vi "CloneMethod.vi"(0 "ClassWriterNative.lvclass":refnum<class "ClassWriterNative.lvclass">, 1 "VIItemRefIn":refnum<vi>, 2 "NewVIPath":path, 3 "LibraryOwners":refnum<vi>[](array[refnum]), 4 "OpenVIWhenDone":bool, 5 "error in (no error)":errorcluster, 7 "ViDescription":string) -> (14 "ClassWriterNative.lvclass":refnum<class "ClassWriterNative.lvclass">, 19 "error out":errorcluster)   [LabVIEW 2020, in "ClassWriterNative.lvclass"]
uses:
  ClassWriterNative.lvclass
  Provider_EndevoGOOP400/EndevoG4ProviderName.ctl
  <vilib>/picture/picture.llb/imagedata.ctl
  <vilib>/Utility/lvfile.llb/NI_FileType.lvlib
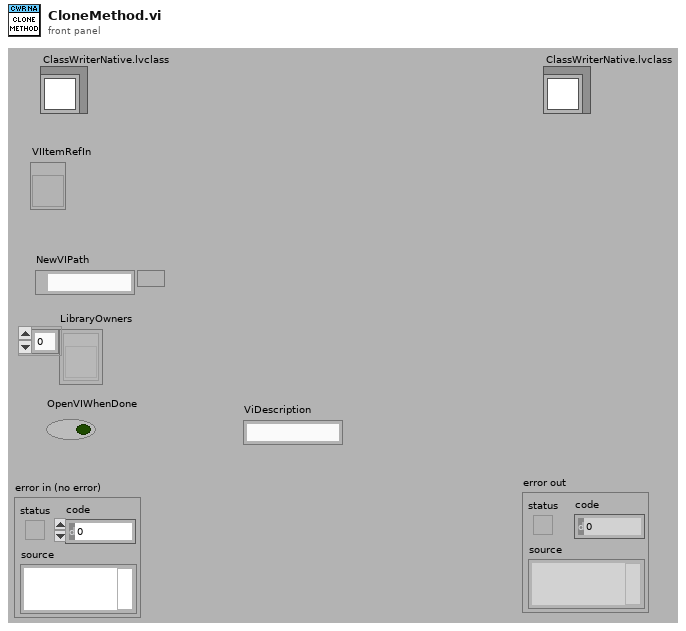
[diagram p1: front panel]
types:
  T1 = cluster{"OrgPath":path, "VIRef":refnum<vi>, "AppRef":refnum<vi>, "NewViRefs":refnum<vi>[], "VIOwner":refnum<vi>, "OrgViLibName":string, "OrgLibFolder":path, "OrgClassPath":path, "OrgClassPathMemberData":path, "FileBackups":string[], "Scope":enum32{"invalid scope", "public", "private", "protected", "community"}}
  T2 = typedef "EndevoG4ProviderName.ctl" = enum16{"EndevoGOOP400"}
  T3 = enum32{"invalid scope", "public", "private", "protected", "community"}
  T4 = typedef "imagedata.ctl" = cluster{"image type":i32, "image depth":i32, "image":u8[], "mask":u8[], "colors":u32[], "Rectangle":cluster{"left":i16, "top":i16, "right":i16, "bottom":i16}}
  T5 = typedef "GOOP400_Options.ctl" = cluster{"FlatFolderStructure":bool}
  T6 = enum32{"invalid scope", "public", "private", "protected", "community"}[]
  T7 = typedef "GDSLvClass_IconSettingsType.ctl" = cluster{"Frame":u32, "Frame thickness":u8, "Header Background":u32, "Header Text":u32, "ColorPublic":u32, "ColorProtected":u32, "ColorPrivate":u32, "Body Text":u32, "ClassBodyIcon":string}
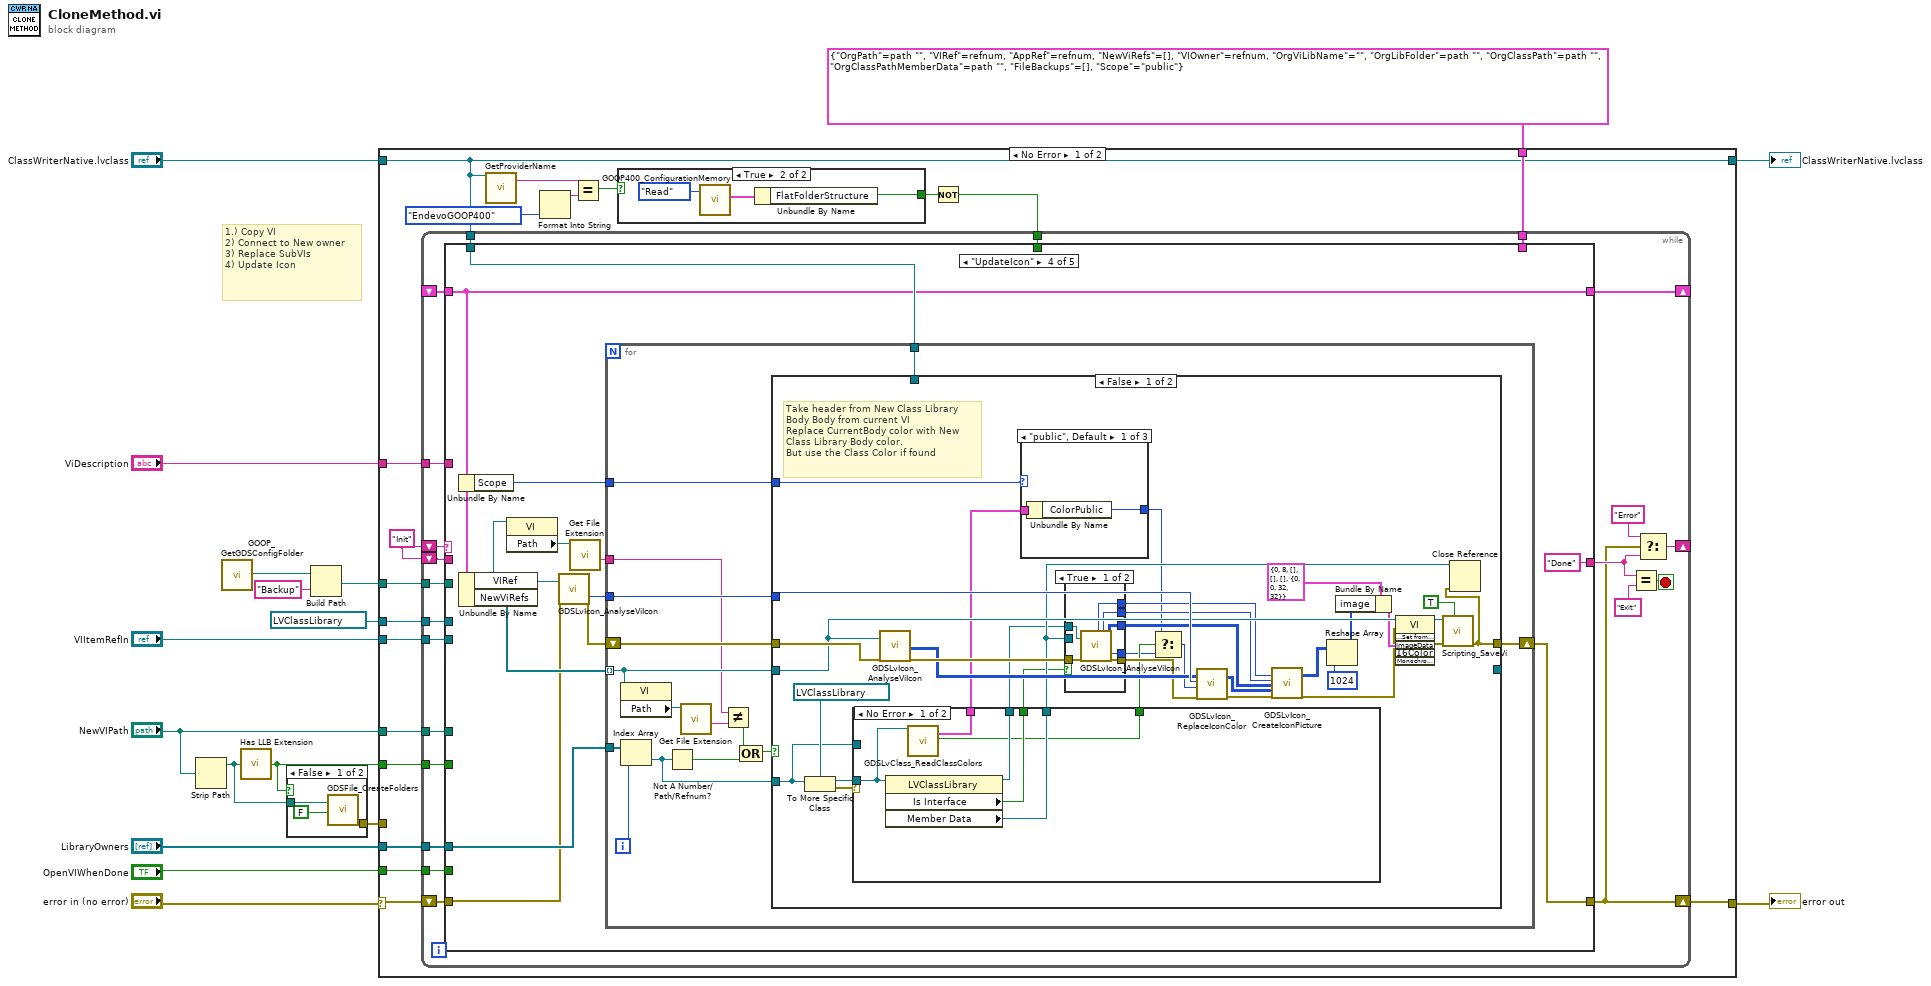
[diagram p0: block diagram]
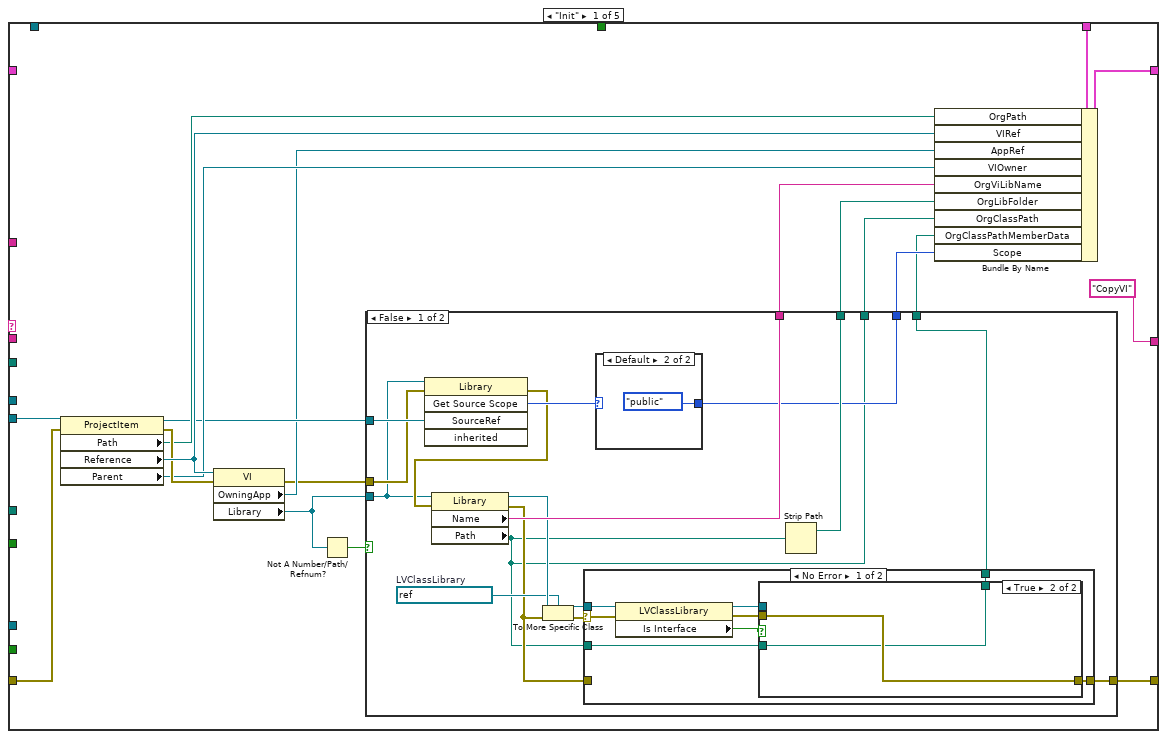
[diagram p4: hidden frame]
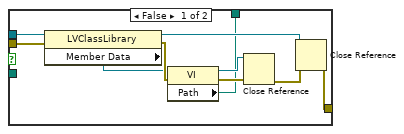
[diagram p6: hidden frame]
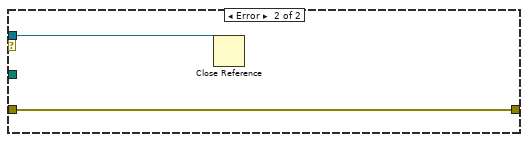
[diagram p7: hidden frame]
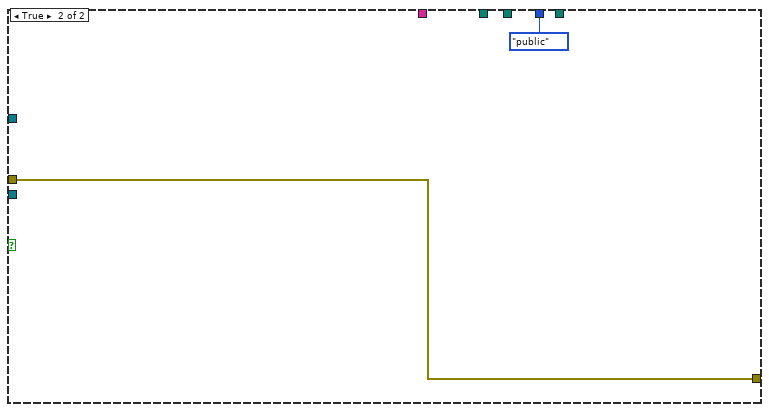
[diagram p8: hidden frame]
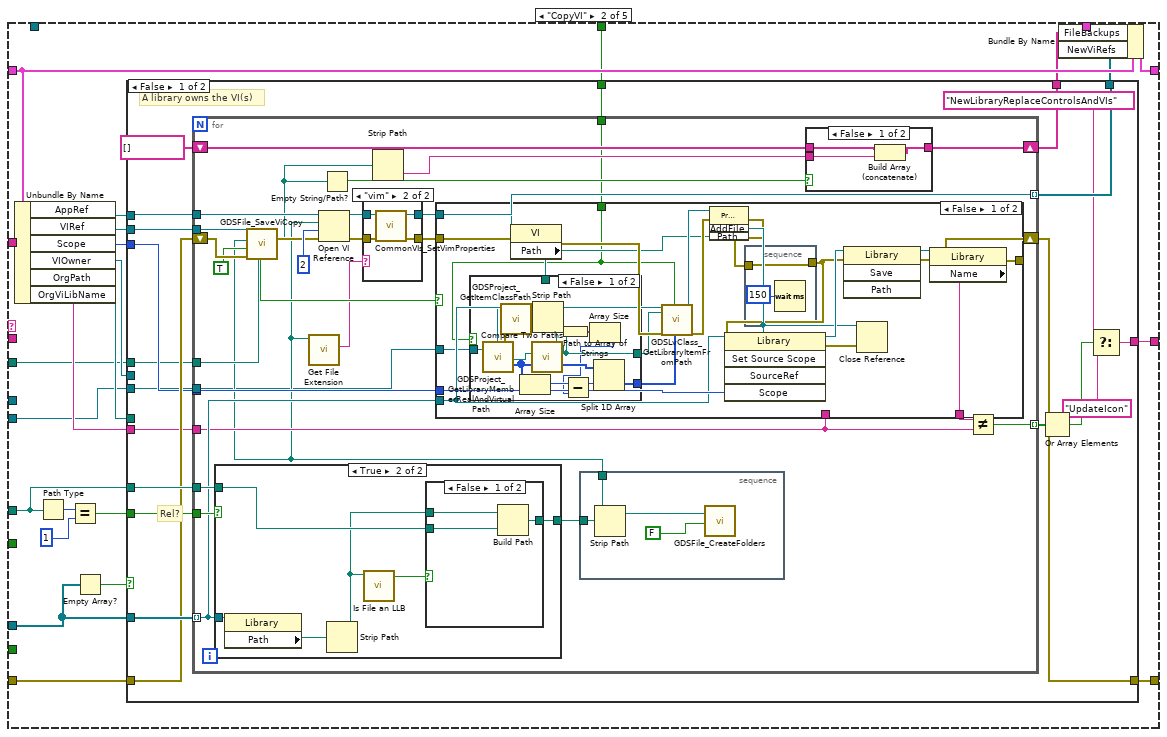
[diagram p9: hidden frame]
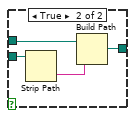
[diagram p15: hidden frame]
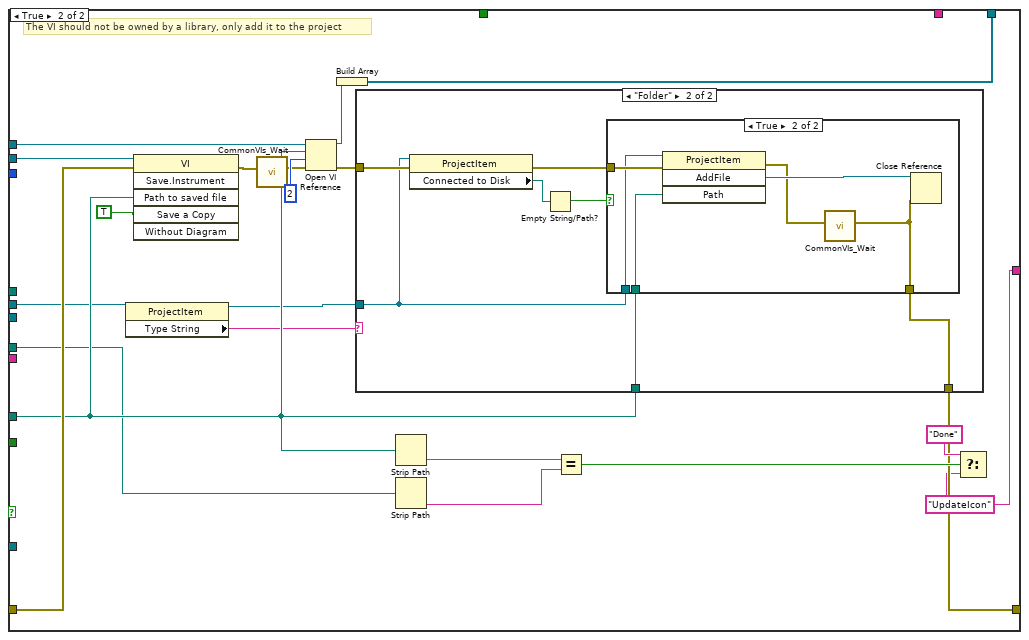
[diagram p16: hidden frame]
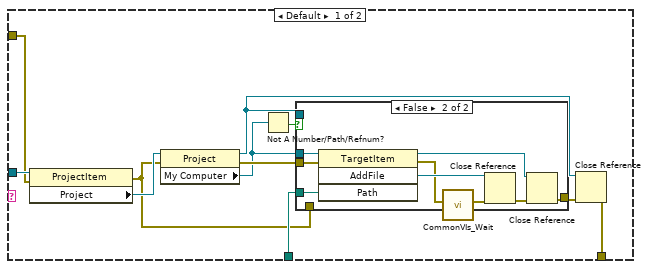
[diagram p17: hidden frame]
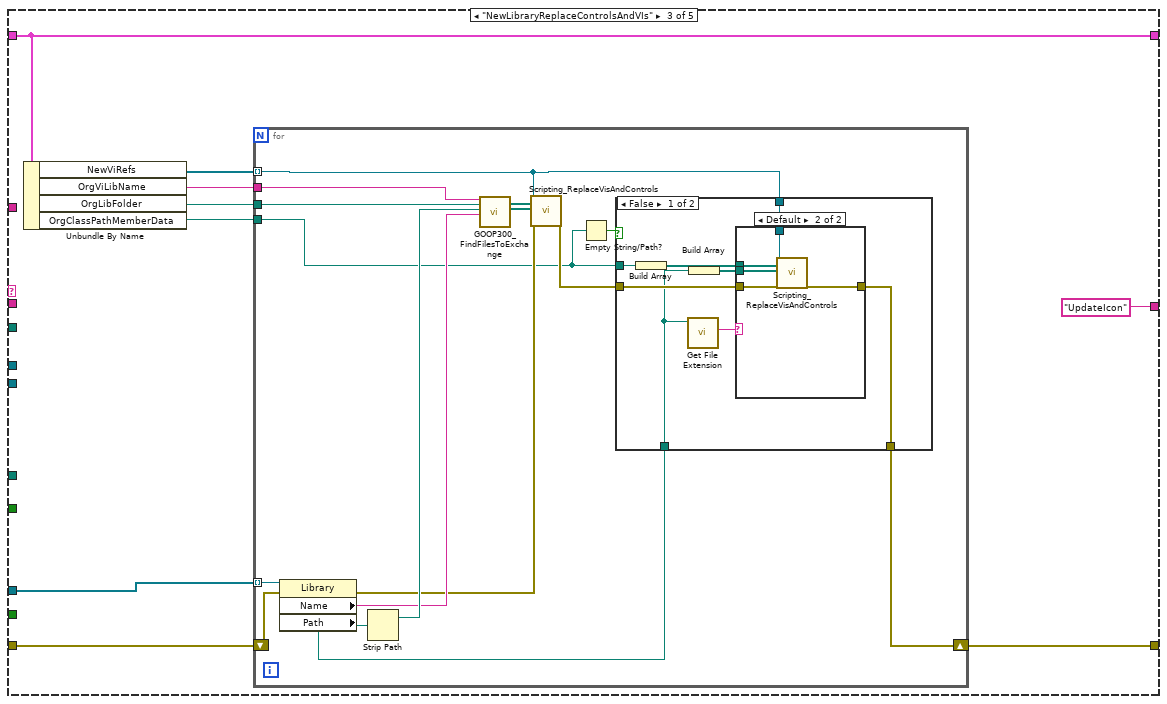
[diagram p20: hidden frame]
diagram:
  # "1.) Copy VI\n2) Connect to New owner\n3) Replace SubVIs\n4) Update Icon"
  n1 = Strip Path(path="NewVIPath") -> (stripped path=w9:path)  [unwired: 1 out]
  n2 = call "GOOP_GetGDSConfigFolder.vi"() -> ("GDSFolderPath"=w8:path)
  n3 = call <vilib>:"Has LLB Extension.vi"("path"=w9) -> ("path to VI library?"=w4:bool)
  n4 = case shown="False" w4 {
    tunnel: w9 -> [w19 _]
    tunnel: [w18 _] -> w5
    frame False {
      n5 = call "GDSFile_CreateFolders.vi"("Path"=w19, "Promt if folder\ndoes not exists?"=FALSE ("Promt if folder\ndoes not exists?")) -> ("error out"=w18:errorcluster)  [unwired: 13 in, 4 out]
    }
    frame True {
    }
  }
  n6 = Build Path(base path=w8, name or relative path="Backup") -> (appended path=w6:path)
  n7 = case shown="No Error" "error in (no error)" {
    selector: "error in (no error)" -> [w39 w529]
    tunnel: [w38 w529] -> w16
    tunnel: "ClassWriterNative.lvclass" -> [w22 w528]
    tunnel: [w22 w528] -> w14
    tunnel: refnum<vi> refnum ("ClassRefOut") -> [w37 _]
    tunnel: "NewVIPath" -> [w36 _]
    tunnel: w4 -> [w35 _]
    tunnel: "LibraryOwners" -> [w34 _]
    tunnel: "VIItemRefIn" -> [w33 _]
    tunnel: w6 -> [w32 _]
    tunnel: w5 -> [_ _]
    tunnel: "OpenVIWhenDone" -> [w31 _]
    tunnel: "ViDescription" -> [w29 _]
    tunnel: T1 {"OrgPath"=path "", "VIRef"=refnum, "AppRef"=refnum, "NewViRefs"=[], "VIOwner"=refnum, "OrgViLibName"="", "OrgLibFolder"=path "", "OrgClassPath"=path "", "OrgClassPathMemberData"=path "", "FileBackups"=[], "Scope"=enum."public"} -> [w28 _]
    frame No Error {
      w30 = "Init"
      n8 = call-dynamic "GetProviderName.vi"("ClassWriterNative in"=w22) -> ("ProviderName"=w24:string)  [unwired: 15 in, 3 out]
      n9 = Format Into String(EndevoG4ProviderName."EndevoGOOP400" ("ProviderName")) -> (resulting string=w23:string)  [unwired: 3 in, 1 out]
      n10 = Equal?(x=w24, y=w23) -> (x = y?=w26:bool)
      n11 = case shown="True" w26 {
        tunnel: [_ w40] -> w27
        frame False {
        }
        frame True {
          n12 = call "GOOP400_ConfigurationMemory.vi"("Action"=enum16{"Read", "Load", "Save"}."Read") -> ("OptionsOut"=w41:T5)  [unwired: 17 in, 1 out]
          n13 = Unbundle By Name(w41) -> ("FlatFolderStructure"=w40:bool)
        }
      }
      n14 = Not(x=w27) -> (.not. x?=w21:bool)
      n15 = while {
        shift-right: [w57] -> w38
        shift-left: w39 -> [w64]
        shift-right: [w62] -> _
        shift-left: w30 -> [w63]
        shift-right: [w56] -> _
        shift-left: _ -> [w55]
        tunnel: w37 -> [w54]
        tunnel: w36 -> [w53]
        tunnel: w35 -> [w52]
        tunnel: w34 -> [w51]
        tunnel: w33 -> [w50]
        tunnel: w32 -> [w49]
        tunnel: w22 -> [w48]
        tunnel: w31 -> [w47]
        shift-left: w30 -> [w46]
        tunnel: w29 -> [w45]
        tunnel: w28 -> [w44]
        tunnel: w21 -> [w43]
        stop <- w61 stop-if-true
        n16 = case shown="\"UpdateIcon\"" w63 {
          tunnel: w64 -> [w84 w143 w322 w367 w486]
          tunnel: [w73 w142 w321 w369 w471] -> w57
          tunnel: ["CopyVI" w139 "UpdateIcon" "Done" "Exit"] -> w58
          tunnel: [w83 w136 w327 w360 w469] -> w56
          tunnel: w55 -> [_ w137 w327 w360 w469]
          tunnel: w54 -> [_ _ _ _ _]
          tunnel: w53 -> [_ w144 _ _ _]
          tunnel: w52 -> [_ _ _ _ _]
          tunnel: w51 -> [_ w141 w325 w368 _]
          tunnel: w50 -> [w80 w127 _ _ _]
          tunnel: w49 -> [_ w130 _ _ w475]
          tunnel: w48 -> [_ _ _ w361 w474]
          tunnel: w47 -> [_ _ _ _ w473]
          tunnel: w46 -> [_ _ _ _ w470]
          tunnel: w45 -> [_ _ _ _ w468]
          tunnel: w44 -> [w65 _ _ _ _]
          tunnel: w43 -> [_ w128 _ _ _]
          frame "Init" {
            n17 = property class="ProjectItem"(reference=w80, error in=w84) -> (reference out=w72:refnum<vi>, error out=w79:errorcluster, "Path"=w75:path, "Reference"=w81:refnum<vi>, "Parent"=w78:refnum<vi>)
            n18 = property class="VI"(reference=w81, error in=w79) -> (error out=w66:errorcluster, "OwningApp"=w68:refnum<vi>, "Library"=w67:refnum<vi>)  [unwired: 1 out]
            n19 = Not A Number/Path/Refnum?(number/path/refnum=w67) -> (NaN/Path/Refnum?=w69:bool)
            n20 = case shown="False" w69 {
              tunnel: [w100 _] -> w77
              tunnel: [w99 _] -> w76
              tunnel: [w85 _] -> w74
              tunnel: [w98 w126] -> w73
              tunnel: w72 -> [w92 _]
              tunnel: [w90 T3."public" ("GetSourceScope")] -> w71
              tunnel: w66 -> [w89 w126]
              tunnel: w67 -> [w87 _]
              tunnel: [w86 _] -> w70
              frame False {
                w96 = refnum<vi> refnum  # LVClassLibrary
                n21 = invoke class="Library" method="Get Source Scope"(reference=w87, error in=w89, "SourceRef"=w92) -> (error out=w88:errorcluster, "GetSourceScope"=w91:T3)  [unwired: 2 in, 3 out]
                n22 = property class="Library"(reference=w87, error in=w88) -> (reference out=w97:refnum<vi>, error out=w94:errorcluster, "Name"=w100:string, "Path"=w85:path)
                n23 = To More Specific Class(target class=w96, reference=w97, error in=w94) -> (specific class reference=w93:refnum<vi>, error out=w95:errorcluster)
                n24 = case shown="No Error" w95 {
                  selector: w95 -> [w108 _]
                  tunnel: [w110 w124] -> w98
                  tunnel: w94 -> [_ w124]
                  tunnel: [w109 _] -> w86
                  tunnel: w93 -> [w107 w123]
                  tunnel: w85 -> [w103 _]
                  frame No Error {
                    n25 = property class="LVClassLibrary"(reference=w107, error in=w108) -> (reference out=w104:refnum<vi>, error out=w105:errorcluster, "Is Interface"=w106:bool)
                    n26 = case shown="True" w106 {
                      tunnel: [w114 w122] -> w110
                      tunnel: [w113 w121] -> w109
                      tunnel: w105 -> [w112 w122]
                      tunnel: w104 -> [w111 _]
                      tunnel: w103 -> [_ w121]
                      frame False {
                        n27 = property class="LVClassLibrary"(reference=w111, error in=w112) -> (reference out=w116:refnum<vi>, error out=w120:errorcluster, "Member Data"=w119:refnum<vi>)
                        n28 = property class="VI"(reference=w119, error in=w120) -> (reference out=w117:refnum<vi>, error out=w118:errorcluster, "Path"=w113:path)
                        n29 = Close Reference(reference=w117, error in (no error)=w118) -> (error out=w115:errorcluster)
                        n30 = Close Reference(reference=w116, error in (no error)=w115) -> (error out=w114:errorcluster)
                      }
                      frame True {
                      }
                    }
                  }
                  frame Error {
                    n31 = Close Reference(reference=w123) -> ()  [unwired: 1 in, 1 out]
                  }
                }
                n32 = case shown="Default" w91 {
                  selector: w91 -> [w101 _]
                  tunnel: [w101 T3."public" ("GetSourceScope")] -> w90
                  frame "private", "protected" {
                  }
                  frame Default {
                  }
                }
                n33 = Strip Path(path=w85) -> (stripped path=w99:path)  [unwired: 1 out]
              }
              frame True {
              }
            }
            n34 = Bundle By Name(cluster=w65, "OrgPath"=w75, "VIRef"=w81, "AppRef"=w68, "VIOwner"=w78, "OrgViLibName"=w77, "OrgLibFolder"=w76, "OrgClassPath"=w74, "OrgClassPathMemberData"=w70, "Scope"=w71) -> (w83:T1)
          }
          frame "CopyVI" {
            n35 = Unbundle By Name(w137) -> ("AppRef"=w138:refnum<vi>, "VIRef"=w145:refnum<vi>, "Scope"=w131:T3, "VIOwner"=w134:refnum<vi>, "OrgPath"=w133:path, "OrgViLibName"=w132:string)
            n36 = Path Type(1:w144) -> (0:w148:i16)
            n37 = Equal?(x=w148, y=i16 1 ("type")) -> (x = y?=w146:bool)
            n38 = Empty Array?(array=w141) -> (empty?=w140:bool)
            n39 = case shown="False" w140 {
              tunnel: w141 -> [w168 _]
              tunnel: w146 -> [w167 _]
              tunnel: w145 -> [w166 w284]
              tunnel: w144 -> [w165 w277]
              tunnel: w143 -> [w164 w278]
              tunnel: [w163 w271] -> w142
              tunnel: [w158 w267] -> w139
              tunnel: w138 -> [w162 w282]
              tunnel: [w161 w279] -> w135
              tunnel: w134 -> [_ w269]
              tunnel: w133 -> [_ w276]
              tunnel: w132 -> [w157 _]
              tunnel: w131 -> [w154 _]
              tunnel: w130 -> [w153 _]
              tunnel: [w151 _] -> w129
              tunnel: w128 -> [w150 _]
              tunnel: w127 -> [w149 _]
              frame False {
                # "A library owns the VI(s)"
                # "Rel?"
                n40 = for {
                  tunnel: w168 -> [w188] mode=indexing
                  tunnel: w167 -> [w197]
                  tunnel: w166 -> [w198]
                  tunnel: w165 -> [w196]
                  shift-right: [w189] -> w163
                  shift-left: w164 -> [w195]
                  tunnel: w162 -> [w192]
                  tunnel: [w172] -> w161 mode=indexing
                  tunnel: w157 -> [w177]
                  tunnel: [w190] -> w156 mode=indexing
                  tunnel: w154 -> [w187]
                  tunnel: w153 -> [w186]
                  shift-right: [w183] -> w151
                  shift-left: string[] [] -> [w184]
                  tunnel: w150 -> [w170]
                  tunnel: w149 -> [w169]
                  n41 = case shown="True" w197 {
                    tunnel: w188 -> [_ w256]
                    tunnel: w196 -> [w250 w254]
                    tunnel: [w250 w252] -> w179
                    frame False {
                    }
                    frame True {
                      n42 = property class="Library"(reference=w256) -> ("Path"=w255:path)  [unwired: 1 in, 2 out]
                      n43 = Strip Path(path=w255) -> (stripped path=w253:path)  [unwired: 1 out]
                      n44 = call <vilib>:"Is File an LLB.vi"("path"=w253) -> ("Is LLB?"=w251:bool)  [unwired: 9 in, 1 out]
                      n45 = case shown="False" w251 {
                        tunnel: w254 -> [w259 w261]
                        tunnel: w253 -> [w258 w262]
                        tunnel: [w257 w263] -> w252
                        frame False {
                          n46 = Build Path(base path=w258, name or relative path=w259) -> (appended path=w257:path)
                        }
                        frame True {
                          n47 = Strip Path(path=w261) -> (name=w260:string)  [unwired: 1 out]
                          n48 = Build Path(base path=w262, name or relative path=w260) -> (appended path=w263:path)
                        }
                      }
                    }
                  }
                  n49 = stacked-sequence {
                    tunnel: w179 -> [w243]
                    tunnel: [w243] -> w176
                    frame #0 {
                      n50 = Strip Path(path=w243) -> (stripped path=w244:path)  [unwired: 1 out]
                      n51 = call "GDSFile_CreateFolders.vi"("Path"=w244, "Promt if folder\ndoes not exists?"=FALSE ("Promt if folder\ndoes not exists?")) -> ()  [unwired: 13 in, 5 out]
                    }
                  }
                  n52 = call "GDSFile_SaveViCopy.vi"("BackupFolder"=w186, "error in"=w195, "OverWirite(False)"=TRUE, "NewCopyPath"=w176, "VIRef"=w198) -> ("error out"=w193:errorcluster, "OverWritten"=w178:bool, "BackupFileName"=w182:path)  [unwired: 4 in]
                  n53 = call <vilib>:"Get File Extension.vi"("file"=w176) -> ("lowercase file extension"=w171:string)  [unwired: 6 in, 4 out]
                  n54 = Open VI Reference(application reference (local)=w192, vi path=w176, options=2, error in (no error)=w193) -> (vi reference=w174:refnum<vi>, error out=w175:errorcluster)  [unwired: 2 in]
                  n55 = Empty String/Path?(string/path=w182) -> (empty?=w185:bool)
                  n56 = case shown="\"vim\"" w171 {
                    tunnel: w175 -> [w199 w204]
                    tunnel: w174 -> [w200 w203]
                    tunnel: [w199 w202] -> w173
                    tunnel: [w200 w201] -> w172
                    frame Default {
                    }
                    frame "vim" {
                      n57 = call "CommonVIs_SetVimProperties.vi"("error in (no error)"=w204, "VIRefIn"=w203) -> ("error out"=w202:errorcluster, "VIRefOut"=w201:refnum<vi>)  [unwired: 8 in]
                    }
                  }
                  n58 = Strip Path(path=w182) -> (name=w181:string)  [unwired: 1 out]
                  n59 = case shown="False" w178 {
                    tunnel: [w220 w242] -> w191
                    tunnel: w173 -> [w219 w241]
                    tunnel: w172 -> [w218 _]
                    tunnel: [w217 w241] -> w189
                    tunnel: w188 -> [w210 _]
                    tunnel: w187 -> [w213 _]
                    tunnel: w177 -> [_ w242]
                    tunnel: w170 -> [w206 _]
                    tunnel: w169 -> [w207 _]
                    frame False {
                      n60 = property class="VI"(reference=w218, error in=w219) -> (error out=w225:errorcluster, "Path"=w209:path)  [unwired: 1 out]
                      n61 = case shown="False" w206 {
                        tunnel: [w231 w238] -> w208
                        tunnel: w209 -> [_ w238]
                        tunnel: w207 -> [w237 _]
                        tunnel: [w226 _] -> w205
                        frame False {
                          n62 = call "GDSProject_GetLibraryMemberRealAndVirtualPath.vi"("LibraryItem"=w237) -> ("LibraryItemVirtualPath"=w233:path, "VirtualFolderScope"=w230:T6, "error out"=w236:errorcluster)  [unwired: 15 in, 1 out]
                          n63 = call "GDSProject_GetItemClassPath.vi"("error in"=w236, "ProjectItemRefIn"=w237) -> ("Path"=w235:path)  [unwired: 4 in, 5 out]
                          n64 = Array Size(array=w230) -> (size(s)=w229:i32)
                          n65 = Strip Path(path=w235) -> (stripped path=w234:path)  [unwired: 1 out]
                          n66 = call <vilib>:"Compare Two Paths.vi"("Path 2"=w233, "Path 1"=w234) -> ("Relative Path from 1 to 2"=w231:path)  [unwired: 6 in, 3 out]
                          n67 = Path to Array of Strings(0:w231) -> (2:w232:string[])  [unwired: 1 out]
                          n68 = Array Size(array=w232) -> (size(s)=w228:i32)
                          n69 = Subtract(x=w229, y=w228) -> (x-y=w227:i32)
                          n70 = Split 1D Array(array=w230, index=w227) -> (second subarray=w226:T6)  [unwired: 1 out]
                        }
                        frame True {
                        }
                      }
                      n71 = call "GDSLvClass_GetLibraryItemFromPath.vi"("Library Refnum In"=w210, "VINames"=w208, "error in (no error)"=w225, "CreateThePhysicalFolderIfPossible(True)"=w206, "VirtualFolderScope"=w205) -> ("Item Refnum Out"=w223:refnum<vi>, "error out"=w224:errorcluster)  [unwired: 13 in]
                      n72 = invoke class="ProjectItem" method="AddFile"(reference=w223, error in=w224, "Path"=w209) -> (error out=w212:errorcluster, "AddFile"=w214:refnum<vi>)  [unwired: 1 in, 2 out]
                      n73 = stacked-sequence {
                        tunnel: [w239] -> w211
                        tunnel: w212 -> [w239]
                        frame #0 {
                          n74 = Wait (ms)(milliseconds to wait=u32 150) -> ()  [unwired: 1 out]
                        }
                      }
                      n75 = invoke class="Library" method="Set Source Scope"(reference=w210, error in=w211, "SourceRef"=w214, "Scope"=w213) -> (reference out=w216:refnum<vi>, error out=w215:errorcluster)  [unwired: 1 in, 3 out]
                      n76 = invoke class="Library" method="Save"(reference=w216, error in=w211) -> (reference out=w222:refnum<vi>, error out=w221:errorcluster)  [unwired: 2 in, 2 out]
                      n77 = Close Reference(reference=w214, error in (no error)=w215) -> ()  [unwired: 1 out]
                      n78 = property class="Library"(reference=w222, error in=w221) -> (error out=w217:errorcluster, "Name"=w220:string)  [unwired: 1 out]
                    }
                    frame True {
                    }
                  }
                  n79 = case shown="False" w185 {
                    tunnel: w184 -> [w248 w249]
                    tunnel: [w247 w249] -> w183
                    tunnel: w181 -> [w246 _]
                    frame False {
                      n80 = Build Array (concatenate)(w248, w246) -> (w247:string[])
                    }
                    frame True {
                    }
                  }
                  n81 = Not Equal?(x=w191, y=w177) -> (x != y?=w190:bool)
                }
                n82 = Or Array Elements(Boolean array=w156) -> (logical OR=w155:bool)
                n83 = Select(t="NewLibraryReplaceControlsAndVIs", s=w155, f="UpdateIcon") -> (s? t:f=w158:string)
              }
              frame True {
                w267 = "UpdateIcon"
                # "The VI should not be owned by a library, only add it to the project"
                n84 = property class="ProjectItem"(reference=w269) -> (reference out=w268:refnum<vi>, "Type String"=w266:string)  [unwired: 1 in, 1 out]
                n85 = invoke class="VI" method="Save.Instrument"(reference=w284, error in=w278, "Path to saved file"=w277, "Save a Copy"=TRUE) -> (error out=w264:errorcluster)  [unwired: 2 in, 5 out]
                n86 = call "CommonVIs_Wait.vi"("error in"=w264) -> ("error out"=w265:errorcluster)  [unwired: 9 in]
                n87 = Open VI Reference(application reference (local)=w282, vi path=w277, options=2, error in (no error)=w265) -> (vi reference=w280:refnum<vi>, error out=w270:errorcluster)  [unwired: 2 in]
                n88 = Build Array(w280) -> (w279:refnum<vi>[])
                n89 = case shown="\"Folder\"" w266 {
                  tunnel: w277 -> [w292 w312]
                  tunnel: [w289 w311] -> w271
                  tunnel: w270 -> [w293 w308]
                  tunnel: w268 -> [w295 w306]
                  frame Default {
                    n90 = property class="ProjectItem"(reference=w295, error in=w293) -> (error out=w285:errorcluster, "Project"=w294:refnum<vi>)  [unwired: 1 out]
                    n91 = property class="Project"(reference=w294, error in=w285) -> (reference out=w286:refnum<vi>, error out=w291:errorcluster, "My Computer"=w288:refnum<vi>)
                    n92 = Not A Number/Path/Refnum?(number/path/refnum=w288) -> (NaN/Path/Refnum?=w287:bool)
                    n93 = case shown="False" w287 {
                      tunnel: w292 -> [_ w305]
                      tunnel: w291 -> [_ w304]
                      tunnel: [w296 w300] -> w290
                      tunnel: w288 -> [_ w297]
                      tunnel: w286 -> [_ _]
                      tunnel: w285 -> [w296 _]
                      frame True {
                      }
                      frame False {
                        n94 = invoke class="TargetItem" method="AddFile"(reference=w297, error in=w304, "Path"=w305) -> (reference out=w301:refnum<vi>, error out=w299:errorcluster, "AddFile"=w303:refnum<vi>)  [unwired: 1 in, 1 out]
                        n95 = call "CommonVIs_Wait.vi"("error in"=w299) -> ("error out"=w298:errorcluster)  [unwired: 9 in]
                        n96 = Close Reference(reference=w303, error in (no error)=w298) -> (error out=w302:errorcluster)
                        n97 = Close Reference(reference=w301, error in (no error)=w302) -> (error out=w300:errorcluster)
                      }
                    }
                    n98 = Close Reference(reference=w286, error in (no error)=w290) -> (error out=w289:errorcluster)
                  }
                  frame "Folder" {
                    n99 = property class="ProjectItem"(reference=w306, error in=w308) -> (error out=w307:errorcluster, "Connected to Disk"=w310:path)  [unwired: 1 out]
                    n100 = Empty String/Path?(string/path=w310) -> (empty?=w309:bool)
                    n101 = case shown="True" w309 {
                      tunnel: w312 -> [_ w319]
                      tunnel: [w313 w314] -> w311
                      tunnel: w307 -> [w313 w317]
                      tunnel: w306 -> [_ w316]
                      frame False {
                      }
                      frame True {
                        n102 = invoke class="ProjectItem" method="AddFile"(reference=w316, error in=w317, "Path"=w319) -> (error out=w315:errorcluster, "AddFile"=w318:refnum<vi>)  [unwired: 1 in, 2 out]
                        n103 = call "CommonVIs_Wait.vi"("error in"=w315) -> ("error out"=w314:errorcluster)  [unwired: 9 in]
                        n104 = Close Reference(reference=w318, error in (no error)=w314) -> ()  [unwired: 1 out]
                      }
                    }
                  }
                }
                n105 = Strip Path(path=w277) -> (name=w275:string)  [unwired: 1 out]
                n106 = Strip Path(path=w276) -> (name=w274:string)  [unwired: 1 out]
                n107 = Equal?(x=w275, y=w274) -> (x = y?=w273:bool)
                n108 = Select(t="Done", s=w273, f=w267) -> ()  [unwired: 1 out]
              }
            }
            n109 = Bundle By Name(cluster=w137, "FileBackups"=w129, "NewViRefs"=w135) -> (w136:T1)
          }
          frame "NewLibraryReplaceControlsAndVIs" {
            n110 = Unbundle By Name(w327) -> ("NewViRefs"=w326:refnum<vi>[], "OrgViLibName"=w323:string, "OrgLibFolder"=w324:path, "OrgClassPathMemberData"=w320:path)
            n111 = for {
              tunnel: w326 -> [w331] mode=indexing
              tunnel: w325 -> [w341] mode=indexing
              tunnel: w324 -> [w343]
              tunnel: w323 -> [w342]
              shift-right: [w333] -> w321
              shift-left: w322 -> [w340]
              tunnel: w320 -> [w330]
              n112 = property class="Library"(reference=w341, error in=w340) -> (error out=w337:errorcluster, "Name"=w338:string, "Path"=w332:path)  [unwired: 1 out]
              n113 = Strip Path(path=w332) -> (stripped path=w339:path)  [unwired: 1 out]
              n114 = call "GOOP300_FindFilesToExchange.vi"("OldClassName(Prefix or suffix for some VIs)"=w342, "OldFolderPath"=w343, "NewFolderPath"=w339, "NewClassName(Prefix or suffix for some VIs)"=w338) -> ("OldFiles"=w336:path[], "NewFileArray"=w335:path[])  [unwired: 14 in]
              n115 = call "Scripting_ReplaceVisAndControls.vi"("ViRef"=w331, "OldVIsAndControls"=w336, "NewVIsAndControls"=w335, "error in (no error)"=w337) -> ("error out"=w334:errorcluster)  [unwired: 14 in, 1 out]
              n116 = Empty String/Path?(string/path=w330) -> (empty?=w329:bool)
              n117 = case shown="False" w329 {
                tunnel: w334 -> [w349 w358]
                tunnel: [w348 w358] -> w333
                tunnel: w332 -> [w347 _]
                tunnel: w331 -> [w345 _]
                tunnel: w330 -> [w344 _]
                frame False {
                  n118 = Build Array(w344) -> (w351:path[])
                  n119 = call <vilib>:"Get File Extension.vi"("file"=w347) -> ("lowercase file extension"=w346:string)  [unwired: 6 in, 4 out]
                  n120 = Build Array(w347) -> (w350:path[])
                  n121 = case shown="Default" w346 {
                    tunnel: w351 -> [_ w357]
                    tunnel: w350 -> [_ w356]
                    tunnel: w345 -> [_ w355]
                    tunnel: w349 -> [w352 w354]
                    tunnel: [w352 w353] -> w348
                    frame "lvlib" {
                    }
                    frame Default {
                      n122 = call "Scripting_ReplaceVisAndControls.vi"("ViRef"=w355, "OldVIsAndControls"=w357, "NewVIsAndControls"=w356, "error in (no error)"=w354) -> ("error out"=w353:errorcluster)  [unwired: 14 in, 1 out]
                    }
                  }
                }
                frame True {
                }
              }
            }
          }
          frame "UpdateIcon" {
            n123 = Unbundle By Name(w360) -> ("Scope"=w359:T3)
            n124 = Unbundle By Name(w360) -> ("VIRef"=w364:refnum<vi>, "NewViRefs"=w370:refnum<vi>[])
            n125 = property class="VI"(reference=w364) -> ("Path"=w363:path)  [unwired: 1 in, 2 out]
            n126 = call "GDSLvIcon_AnalyseViIcon.vi"("ViRef/LvCLassRef/LvLibRef/ViPath/2D_Image"=w364, "error in (no error)"=w367) -> ("BodyBkColor"=w365:u32, "error out"=w366:errorcluster)  [unwired: 5 in, 11 out]
            n127 = call <vilib>:"Get File Extension.vi"("file"=w363) -> ("filename without extension"=w362:string)  [unwired: 6 in, 4 out]
            n128 = for {
              tunnel: w370 -> [w379] mode=indexing
              shift-right: [w385] -> w369
              shift-left: w366 -> [w386]
              tunnel: w368 -> [w384]
              tunnel: w365 -> [w380]
              tunnel: w362 -> [w376]
              tunnel: w361 -> [w373]
              tunnel: w359 -> [w372]
              i -> [w383]
              n129 = property class="VI"(reference=w379) -> ("Path"=w378:path)  [unwired: 1 in, 2 out]
              n130 = Index Array(array=w384, index=w383) -> (element=w374:refnum<vi>)
              n131 = Not A Number/Path/Refnum?(number/path/refnum=w374) -> (NaN/Path/Refnum?=w382:bool)
              n132 = call <vilib>:"Get File Extension.vi"("file"=w378) -> ("filename without extension"=w377:string)  [unwired: 6 in, 4 out]
              n133 = Not Equal?(x=w376, y=w377) -> (x != y?=w375:bool)
              n134 = Compound Arithmetic op=OR(w375, w382) -> (w381:bool)
              n135 = case shown="False" w381 {
                tunnel: w379 -> [w413 w464]
                tunnel: w386 -> [w415 w459]
                tunnel: [w416 w457] -> w385
                tunnel: w380 -> [w420 _]
                tunnel: [_ w463] -> _
                tunnel: w374 -> [w411 _]
                tunnel: w373 -> [_ w455]
                tunnel: w372 -> [w389 _]
                frame False {
                  # "Take header from New Class Library\nBody Body from current VI\nReplace CurrentBody color with New\nClass Library Body color.\nBut use the Class Color if found"
                  n136 = To More Specific Class(target class=refnum<vi> refnum ("Class Refnum In"), reference=w411) -> (specific class reference=w418:refnum<vi>, error out=w417:errorcluster)  [unwired: 1 in]
                  n137 = case shown="No Error" w417 {
                    tunnel: w418 -> [w443 _]
                    tunnel: [w446 w450] -> w410
                    tunnel: w411 -> [_ w447]
                    tunnel: [w445 _] -> w409
                    tunnel: [w444 _] -> w408
                    tunnel: [w442 _] -> w392
                    tunnel: [w441 _] -> w388
                    frame No Error {
                      n138 = property class="LVClassLibrary"(reference=w443) -> (reference out=w444:refnum<vi>, "Is Interface"=w445:bool, "Member Data"=w446:refnum<vi>)  [unwired: 1 in, 1 out]
                      n139 = call "GDSLvClass_ReadClassColors.vi"("Library Refnum"=w443) -> ("LvClassIconSettings"=w441:T7, "LvClassIconSettingsFound"=w442:bool)  [unwired: 13 in, 4 out]
                    }
                    frame Error {
                      n140 = invoke class="Library" method="Get All Descendents"(reference=w447, "Type"="VI") -> ("All Descendents"=w448:refnum<vi>[])  [unwired: 5 in, 6 out]
                      n141 = Index Array(array=w448) -> (element=w451:refnum<vi>)  [unwired: 1 in]
                      n142 = property class="ProjectItem"(reference=w451) -> (error out=w449:errorcluster, "Reference"=w450:refnum<vi>)  [unwired: 1 in, 1 out]
                      n143 = for {
                        tunnel: w449 -> [w454]
                        tunnel: w448 -> [w453] mode=indexing
                        n144 = Close Reference(reference=w453, error in (no error)=w454) -> ()  [unwired: 1 out]
                      }
                    }
                  }
                  n145 = call "GDSLvIcon_AnalyseViIcon.vi"("ViRef/LvCLassRef/LvLibRef/ViPath/2D_Image"=w413, "error in (no error)"=w415) -> ("BodyIcon"=w412:u8[][], "error out"=w414:errorcluster)  [unwired: 5 in, 11 out]
                  n146 = case shown="\"public\", Default" w389 {
                    tunnel: w388 -> [w422 w424 w426]
                    tunnel: [w421 w423 w425] -> w387
                    frame "public", Default {
                      n147 = Unbundle By Name(w422) -> ("ColorPublic"=w421:u32)
                    }
                    frame "private" {
                      n148 = Unbundle By Name(w424) -> ("ColorPrivate"=w423:u32)
                    }
                    frame "protected" {
                      n149 = Unbundle By Name(w426) -> ("ColorProtected"=w425:u32)
                    }
                  }
                  n150 = case shown="True" w409 {
                    tunnel: [w433 w440] -> w407
                    tunnel: [w432 w439] -> w395
                    tunnel: [w431 w438] -> w394
                    tunnel: [w430 w437] -> w393
                    tunnel: [w429 w436] -> w391
                    tunnel: w414 -> [w428 w435]
                    tunnel: w410 -> [_ w434]
                    tunnel: w408 -> [w427 _]
                    frame True {
                      n151 = call "GDSLvIcon_AnalyseViIcon.vi"("ViRef/LvCLassRef/LvLibRef/ViPath/2D_Image"=w427, "error in (no error)"=w428) -> ("FrameColor"=w431:u32, "FrameThickness(1)"=w430:u32, "HeaderIcon"=w432:u8[][], "BodyBkColor"=w429:u32, "error out"=w433:errorcluster)  [unwired: 5 in, 8 out]
                    }
                    frame False {
                      n152 = call "GDSLvIcon_AnalyseViIcon.vi"("ViRef/LvCLassRef/LvLibRef/ViPath/2D_Image"=w434, "error in (no error)"=w435) -> ("FrameColor"=w438:u32, "FrameThickness(1)"=w437:u32, "HeaderIcon"=w439:u8[][], "BodyBkColor"=w436:u32, "error out"=w440:errorcluster)  [unwired: 5 in, 8 out]
                    }
                  }
                  n153 = Select(t=w387, s=w392, f=w391) -> (s? t:f=w390:u32)
                  n154 = call "GDSLvIcon_ReplaceIconColor.vi"("IconIn"=w412, "OldColor"=w420, "NewColor"=w390, "error in (no error)"=w407) -> ("IconOut"=w399:u8[][], "error out"=w401:errorcluster)  [unwired: 14 in]
                  n155 = call "GDSLvIcon_CreateIconPicture.vi"("FrameColor"=w394, "FrameThickness(1)"=w393, "HeaderIconIn"=w395, "BodyIconIn"=w399, "error in (no error)"=w401) -> ("WholeIconOut"=w404:u8[][], "error out"=w400:errorcluster)  [unwired: 9 in, 4 out]
                  n156 = Reshape Array(w404, 1024 ("dimension size")) -> (w402:u8[])
                  n157 = Bundle By Name(cluster=T4 {"image type"=0, "image depth"=8, "image"=[], "mask"=[], "colors"=[], "Rectangle"={"left"=0, "top"=0, "right"=32, "bottom"=32}} ("image data"), "image"=w402) -> (w405:T4)
                  n158 = invoke class="VI" method="VI Icon.Set from Image Data"(reference=w413, error in=w400, "ImageData"=w405) -> (reference out=w397:refnum<vi>, error out=w398:errorcluster)  [unwired: 3 in, 4 out]
                  n159 = call "Scripting_SaveVi.vi"("ForceResaving(False)"=TRUE, "error in (no error)"=w398, "VIRefToSaveIn"=w397) -> ("error out"=w416:errorcluster)  [unwired: 7 in, 1 out]
                  n160 = Close Reference(reference=w410, error in (no error)=w416) -> ()  [unwired: 1 out]
                }
                frame True {
                  n161 = call-dynamic "ProgressWindow.vi"("ClassWriter in"=w455, "Message(Exit)"="Hide", "error in (no error)"=w459) -> ("ClassWriter out"=w461:refnum<class "ClassWriterNative.lvclass">, "error out"=w458:errorcluster)  [unwired: 15 in]
                  n162 = stacked-sequence {
                    tunnel: w464 -> [w465]
                    tunnel: w458 -> [w467]
                    tunnel: [w466] -> w456
                    tunnel: [w465] -> w463
                    frame #0 {
                      n163 = call "GDSIconEditor_CreateVIIcon.vi"("ViRef(IgnoreIfNotWired)"=w465, "error in (no error)"=w467) -> ("error out"=w466:errorcluster)  [unwired: 9 in]
                    }
                  }
                  n164 = call-dynamic "ProgressWindow.vi"("ClassWriter in"=w461, "Message(Exit)"="UnHide", "error in (no error)"=w456) -> ("error out"=w457:errorcluster)  [unwired: 15 in, 1 out]
                }
              }
            }
          }
          frame "Done", "Error", Default {
            n165 = Unbundle By Name(w469) -> ("FileBackups"=w477:string[], "VIRef"=w479:refnum<vi>, "NewViRefs"=w487:refnum<vi>[], "VIOwner"=w484:refnum<vi>, "AppRef"=w482:refnum<vi>)
            n166 = for {
              tunnel: w487 -> [w513] mode=indexing
              shift-right: [w512] -> w481
              shift-left: w486 -> [w505]
              tunnel: w473 -> [w507]
              tunnel: w468 -> [w503]
              n167 = case shown="Default" w503 {
                selector: w503 -> [_ w516]
                tunnel: w513 -> [w515 w520]
                tunnel: [w515 w519] -> w506
                tunnel: w505 -> [w514 w518]
                tunnel: [w514 w517] -> w504
                frame "" {
                }
                frame Default {
                  n168 = property class="VI"(reference=w520, error in=w518, "Description"=w516) -> (reference out=w519:refnum<vi>, error out=w517:errorcluster)
                }
              }
              n169 = invoke class="VI" method="Save.Instrument"(reference=w506, error in=w504) -> (reference out=w511:refnum<vi>, error out=w509:errorcluster)  [unwired: 4 in, 4 out]
              n170 = case shown="True" w507 {
                tunnel: w511 -> [w522 w527]
                tunnel: [w521 w525] -> w510
                tunnel: w509 -> [w521 w524]
                tunnel: [w522 w523] -> w508
                frame False {
                }
                frame True {
                  n171 = property class="VI"(reference=w527, error in=w524, "Front Panel.Open"=TRUE ("Front Panel Window:Open")) -> (reference out=w523:refnum<vi>, error out=w525:errorcluster)
                }
              }
              n172 = Close Reference(reference=w508, error in (no error)=w510) -> (error out=w512:errorcluster)
            }
            n173 = Empty Array?(array=w477) -> (empty?=w478:bool)
            n174 = Close Reference(reference=w479, error in (no error)=w481) -> (error out=w480:errorcluster)
            n175 = Close Reference(reference=w484, error in (no error)=w480) -> (error out=w483:errorcluster)
            n176 = Array Size(array=w477) -> (size(s)=w476:i32)
            n177 = Close Reference(reference=w482, error in (no error)=w483) -> (error out=w472:errorcluster)
            n178 = case shown="False" w478 {
              tunnel: w476 -> [w497 _]
              tunnel: w475 -> [w496 _]
              tunnel: w472 -> [w493 _]
              tunnel: w474 -> [w488 _]
              frame False {
                n179 = case shown="2, Default" w497 {
                  tunnel: ["%d file has been overwritten.\nA backup of this could be found here:\n%s" ("message") "%d files have been overwritten.\nA backup of these could be found here:\n%s" ("message")] -> w498
                  frame 1 {
                  }
                  frame 2, Default {
                  }
                }
                n180 = call-dynamic "ProgressWindow.vi"("ClassWriter in"=w488, "Message(Exit)"="Hide", "error in (no error)"=w493) -> ("ClassWriter out"=w490:refnum<class "ClassWriterNative.lvclass">, "error out"=w492:errorcluster)  [unwired: 15 in]
                n181 = Format Into String(format string=w498, w497, w496) -> (resulting string=w495:string)  [unwired: 2 in, 1 out]
                n182 = stacked-sequence {
                  tunnel: w495 -> [w500]
                  tunnel: [w499] -> w489
                  tunnel: w490 -> [w499]
                  frame #0 {
                    n183 = One Button Dialog(message=w500) -> ()  [unwired: 1 in, 1 out]
                  }
                }
                n184 = call-dynamic "ProgressWindow.vi"("ClassWriter in"=w489, "Message(Exit)"="UnHide", "error in (no error)"=w492) -> ()  [unwired: 15 in, 2 out]
              }
              frame True {
              }
            }
            n185 = call "GDSError_LogErrorInformation.vi"("State"=w470, "LocalVariableData"=w469, "error in (no error)"=w472) -> ("error out"=w471:errorcluster)  [unwired: 16 in]
          }
        }
        n186 = Equal?(x=w58, y="Exit") -> (x = y?=w61:bool)
        n187 = Select(t="Error", s=w57, f=w58) -> (s? t:f=w62:string)
      }
    }
    frame Error {
    }
  }
  "ClassWriterNative.lvclass" <- w14
  "error out" <- w16
